vi "Tool.vi"() -> ()   [LabVIEW 2015]
uses:
  user32.dll
panel:
  in  "Tab":enum32{"MD5 Tool"}(tab)
  in  "Path":path caption="File Path"
  out "MD5 Checksum":string caption="String"
  in  "OK":bool
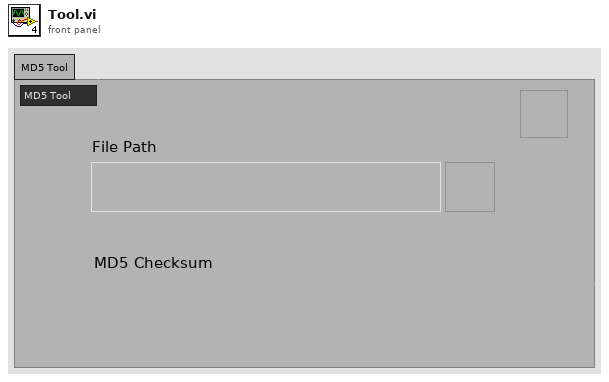
[diagram p1: front panel]
types:
  T1 = enum32{"invalid app kind", "Development System", "Run Time System", "Student Edition", "Embedded LabVIEW", "Evaluation", "Custom"}
  T2 = enum32{"Invalid", "Standard", "Closed", "Hidden", "Minimized", "Maximized"}
  T3 = cluster{"Core":cluster{"Current VI Reference":refnum<vi>, "Close Panel on Exit?":bool}, "Your Boolean data":bool, "Your string data":string}
  T4 = cluster{"Current VI Reference":refnum<vi>, "Close Panel on Exit?":bool}
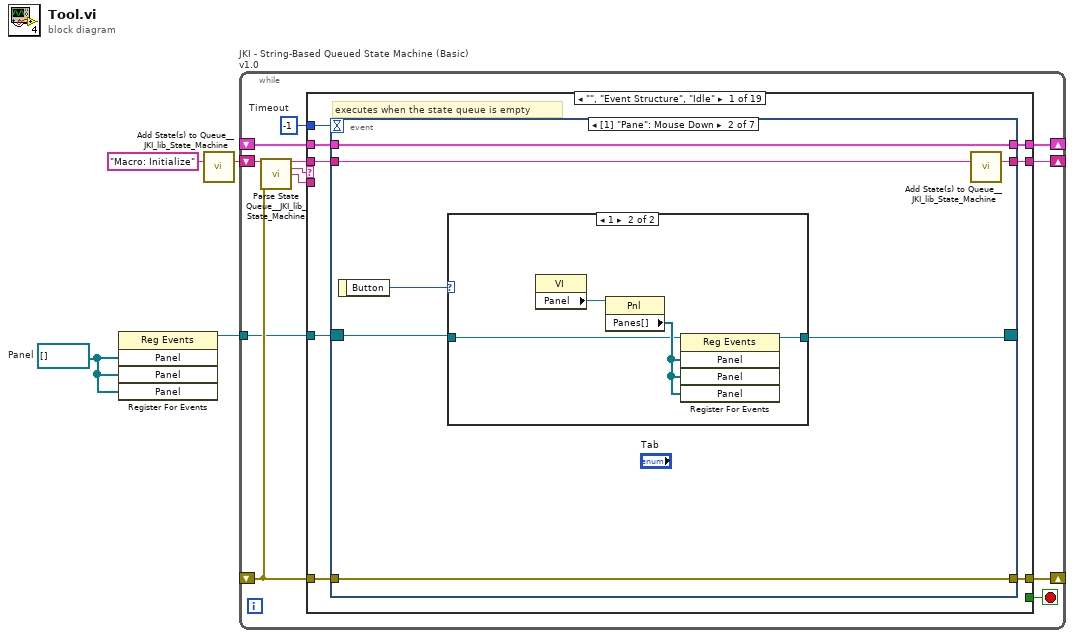
[diagram p0: block diagram]
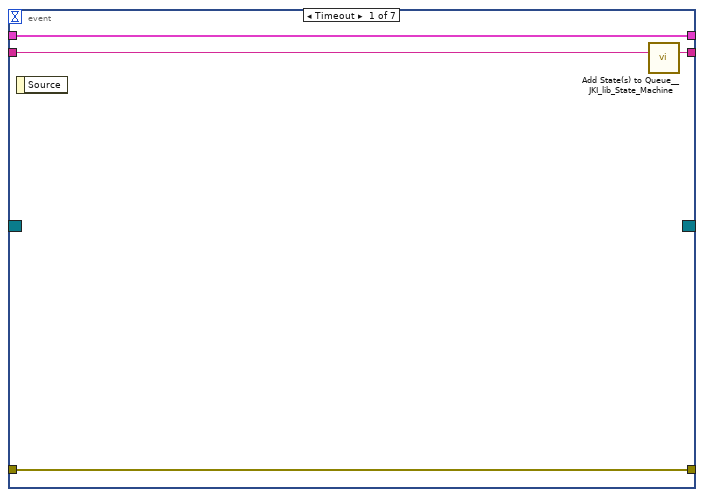
[diagram p2: hidden frame]
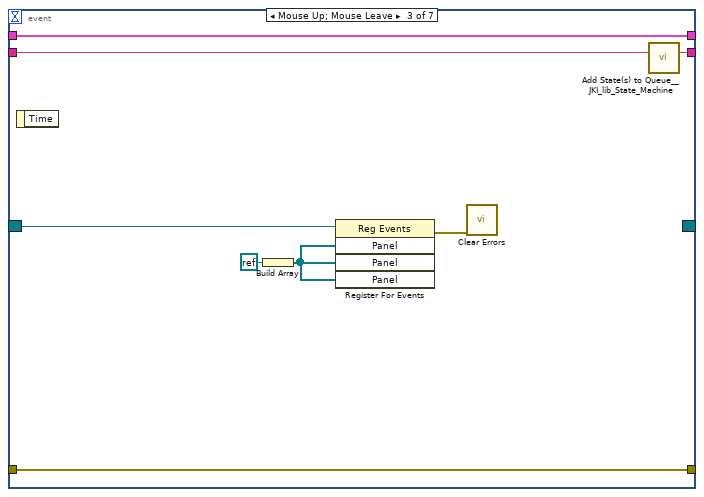
[diagram p4: hidden frame]
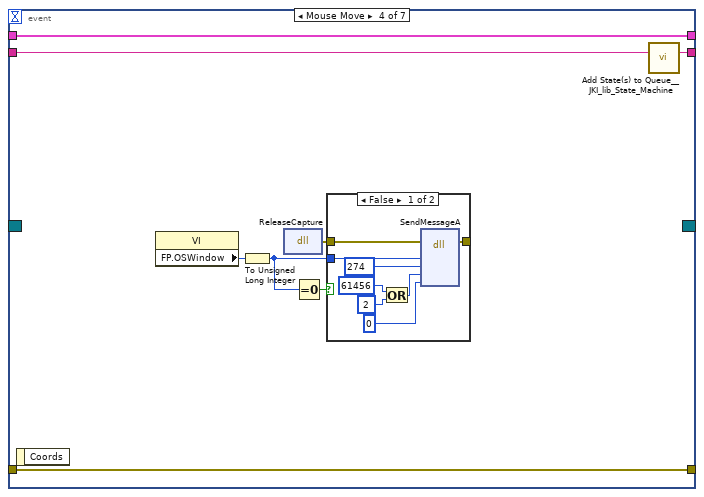
[diagram p5: hidden frame]
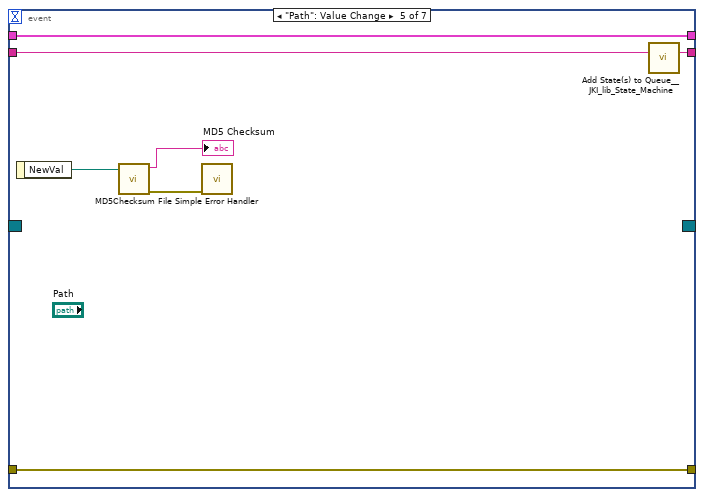
[diagram p7: hidden frame]
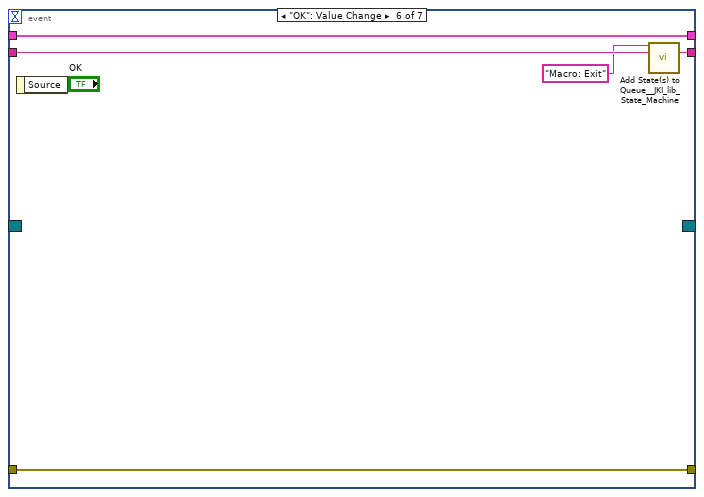
[diagram p8: hidden frame]
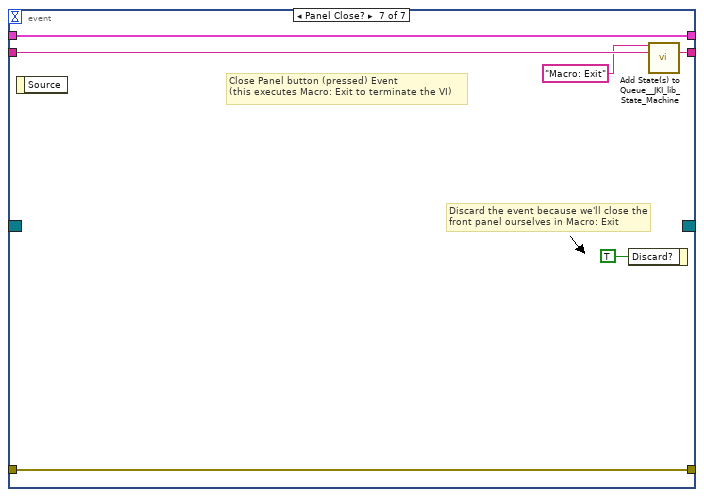
[diagram p9: hidden frame]
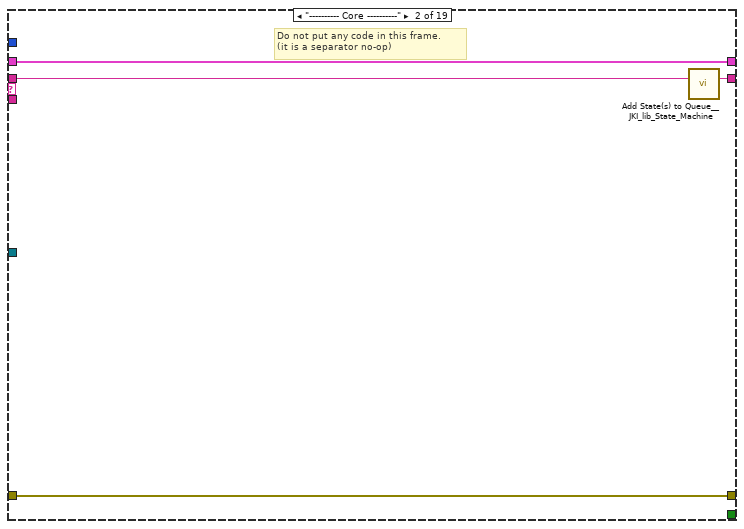
[diagram p10: hidden frame]
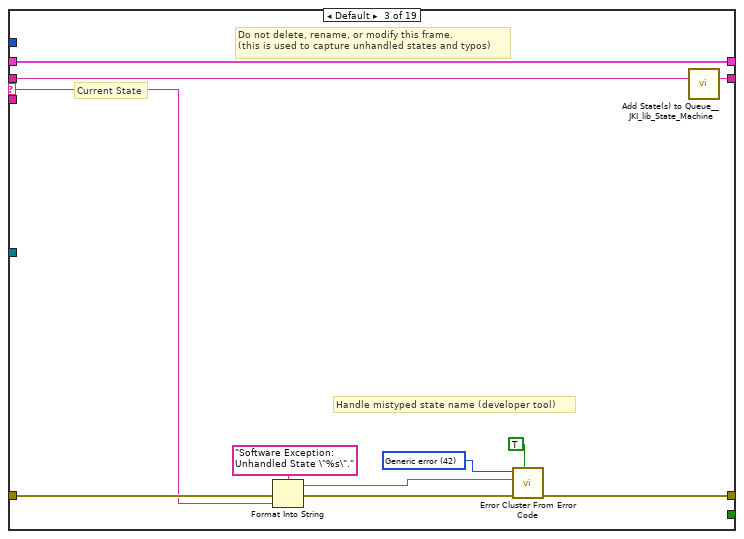
[diagram p11: hidden frame]
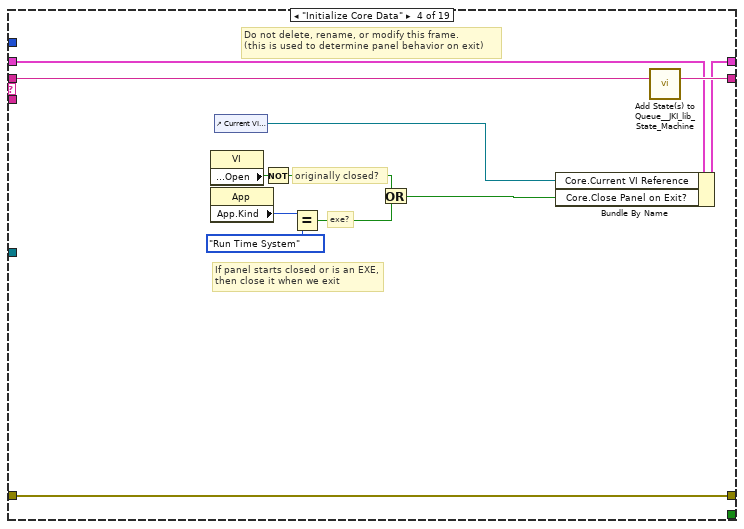
[diagram p12: hidden frame]
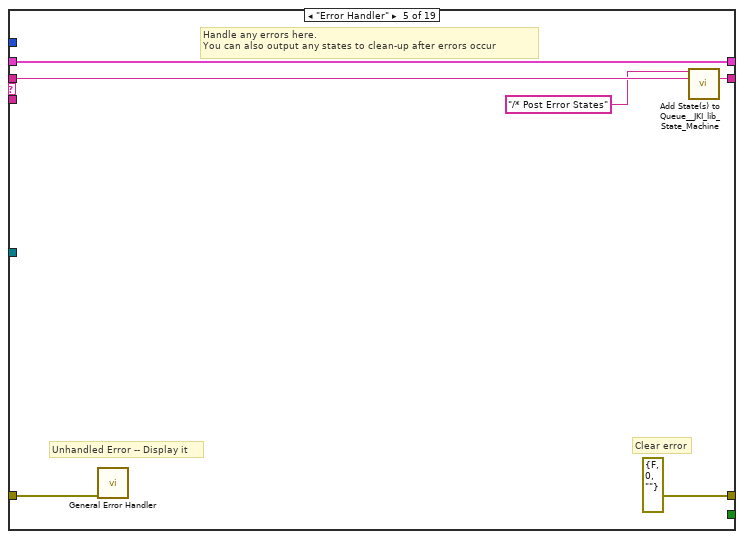
[diagram p13: hidden frame]
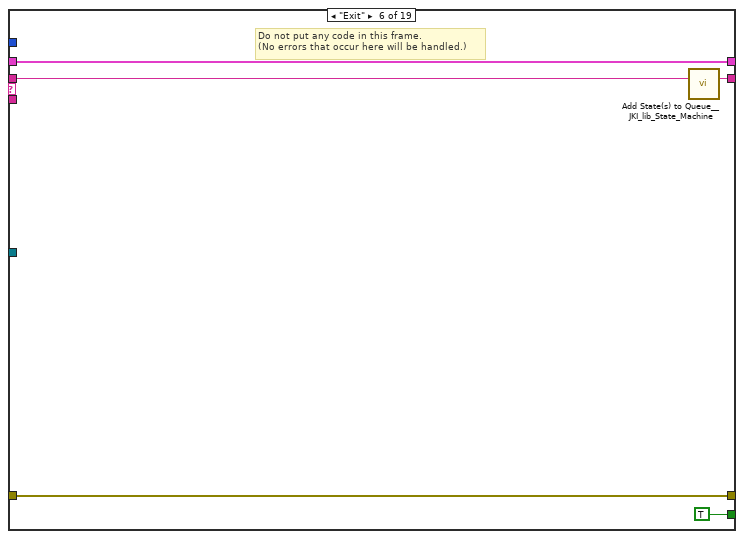
[diagram p14: hidden frame]
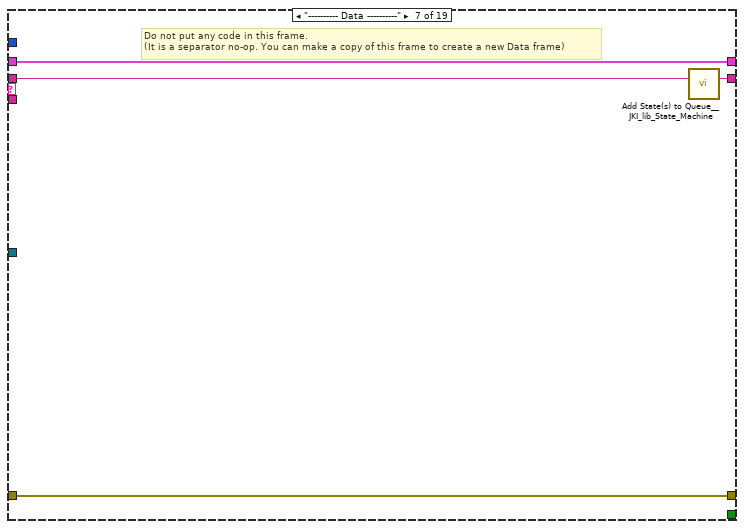
[diagram p15: hidden frame]
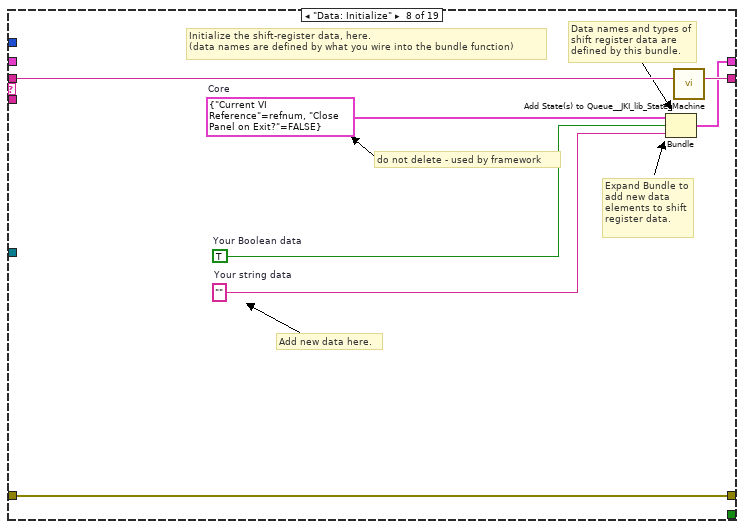
[diagram p16: hidden frame]
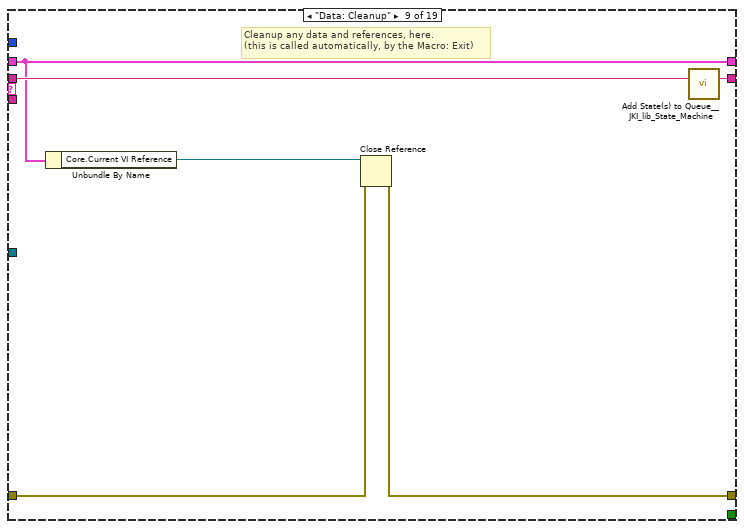
[diagram p17: hidden frame]
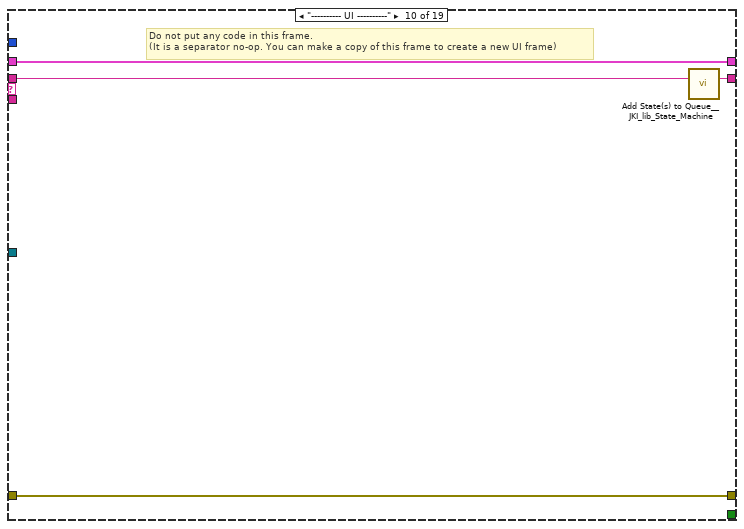
[diagram p18: hidden frame]
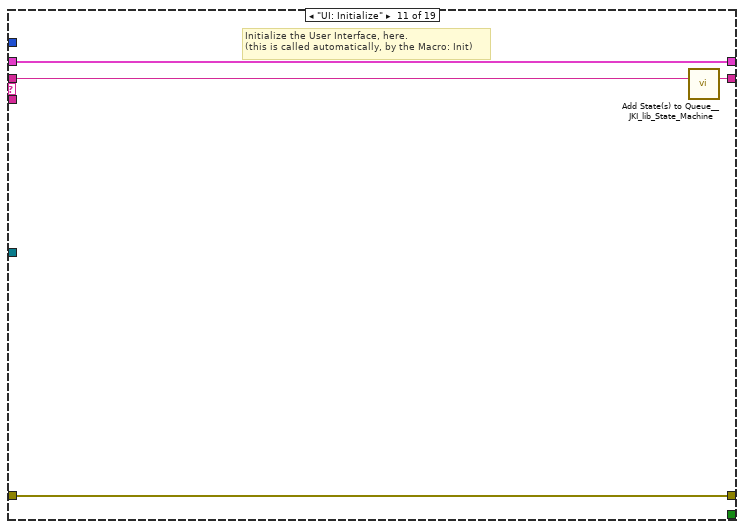
[diagram p19: hidden frame]
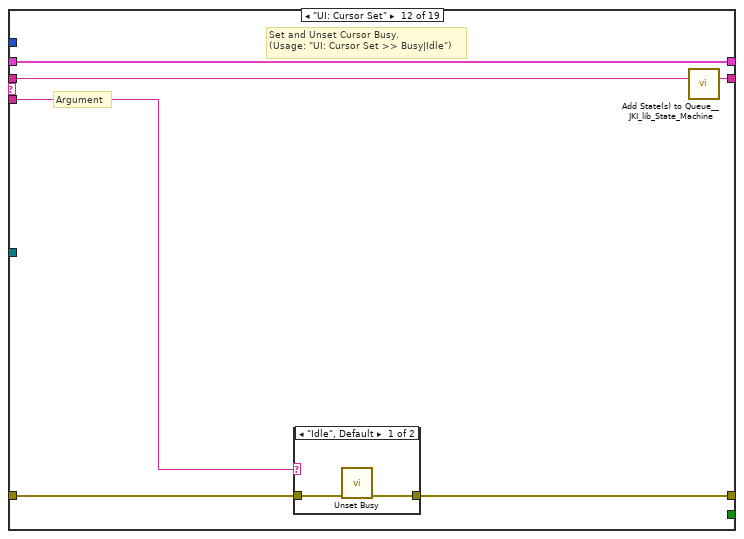
[diagram p20: hidden frame]
diagram:
  w2 = refnum<vi>[] []  # Panel
  n1 = register-events(w2, w2, w2) -> (reference out=w1:refnum<event-registration>)  [unwired: 2 in, 1 out]
  n2 = call <vilib>:"Add State(s) to Queue__JKI_lib_State_Machine.vi"("State(s) in (\"\")"="Macro: Initialize") -> ("States Out"=w4:string)  [unwired: 14 in]
  n3 = while "JKI - String-Based Queued State Machine (Basic) v1.0" {
    shift-right: [w9] -> _
    shift-left: _ -> [w8]
    shift-right: [w12] -> _
    shift-left: _ -> [w6]
    shift-right: [w11] -> _
    shift-left: w4 -> [w13]
    tunnel: w1 -> [w5]
    stop <- w10 stop-if-true
    w7 = -1  # Timeout
    n4 = call <vilib>:"Parse State Queue__JKI_lib_State_Machine.vi"("State Queue"=w13, "Error In (no error)"=w6) -> ("Remaining States"=w15:string, "Current State"=w16:string, "Arguments"=w14:string)  [unwired: 10 in, 1 out]
    n5 = case shown="\"\", \"Event Structure\", \"Idle\"" w16 {
      selector: w16 -> [_ _ w88 _ _ _ _ _ _ _ _ _ _ _ _ _ _ _ _]
      tunnel: w15 -> [w24 w87 w92 w110 w116 w121 w125 w132 w138 w142 w146 w152 w163 w189 w194 w204 w208 w212 w216]
      tunnel: w14 -> [_ _ _ _ _ _ _ _ _ _ _ w147 w157 _ _ _ _ _ _]
      tunnel: w8 -> [w22 w84 w90 w101 w113 w119 w122 _ w133 w139 w144 w150 w159 w186 w191 w201 w205 w209 w213]
      tunnel: [w21 w85 w94 w107 errorcluster {"status"=FALSE, "code"=0, "source"=""} ("error out") w118 w123 w129 w134 w140 w143 w148 w160 w187 w192 w202 w206 w210 w214] -> w12
      tunnel: w6 -> [w20 w85 w93 w107 w112 w118 w123 w129 w135 w140 w143 w149 w161 w187 w192 w202 w206 w210 w214]
      tunnel: [w23 w86 w91 w109 w115 w120 w124 w131 w137 w141 w145 w151 w162 w188 w193 w203 w207 w211 w215] -> w11
      tunnel: [_ _ _ _ _ TRUE _ _ _ _ _ _ _ _ _ _ _ _ _] -> w10
      tunnel: [w19 w84 w90 w108 w113 w119 w122 w130 w133 w139 w144 w150 w159 w186 w191 w201 w205 w209 w213] -> w9
      tunnel: w7 -> [w18 _ _ _ _ _ _ _ _ _ _ _ _ _ _ _ _ _ _]
      tunnel: w5 -> [w17 _ _ _ _ _ _ _ _ _ _ _ _ _ _ _ _ _ _]
      frame "", "Event Structure", "Idle" {
        # "executes when the state queue is empty"
        n6 = event shown="[1] \"Pane\": Mouse Down" {
          selector: w17 -> [_ w31 w41 _ _ _ _]
          dyn-events: [_ w29 _ _ _ _ _] -> _
          timeout: w18 -> [_ _ _ _ _ _ _]
          tunnel: w24 -> [w28 w35 w48 w56 w72 w77 w83]
          tunnel: [w27 w34 w47 w55 w71 w76 w82] -> w23
          tunnel: w22 -> [w25 w32 w45 w53 w69 w74 w80]
          tunnel: [w26 w33 w46 w54 w70 w75 w81] -> w21
          tunnel: w20 -> [w26 w33 w46 w54 w70 w75 w81]
          tunnel: [w25 w32 w45 w53 w69 w74 w80] -> w19
          event Timeout {
            n7 = event-data() -> ()  [unwired: 1 in, 1 out]
            n8 = call <vilib>:"Add State(s) to Queue__JKI_lib_State_Machine.vi"("State(s) in (\"\")"=w28) -> ("States Out"=w27:string)  [unwired: 14 in]
          }
          event Mouse Down {
            n9 = event-data() -> ("Button"=w30:u16)  [unwired: 1 in]
            n10 = case shown="1" w30 {
              tunnel: [w36 w37] -> w29
              tunnel: w31 -> [w36 w38]
              frame 0, Default {
              }
              frame 1 {
                n11 = property class="VI"() -> ("Panel"=w40:refnum<vi>)  [unwired: 2 in, 2 out]
                n12 = property class="Pnl"(reference=w40) -> ("Panes[]"=w39:refnum<vi>[])  [unwired: 1 in, 2 out]
                n13 = register-events(reference=w38, w39, w39, w39) -> (reference out=w37:refnum<event-registration>)  [unwired: 1 in, 1 out]
              }
            }
            n14 = call <vilib>:"Add State(s) to Queue__JKI_lib_State_Machine.vi"("State(s) in (\"\")"=w35) -> ("States Out"=w34:string)  [unwired: 14 in]
          }
          event Mouse Up; Mouse Leave {
            n15 = event-data() -> ()  [unwired: 1 in, 1 out]
            n16 = Build Array(refnum<k0> refnum) -> (w42:refnum<k0>[])
            n17 = register-events(reference=w41, w42, w42, w42) -> (error out=w43:errorcluster)  [unwired: 1 in, 1 out]
            n18 = call <vilib>:"Clear Errors.vi"("error in (no error)"=w43) -> ()  [unwired: 5 in, 2 out]
            n19 = call <vilib>:"Add State(s) to Queue__JKI_lib_State_Machine.vi"("State(s) in (\"\")"=w48) -> ("States Out"=w47:string)  [unwired: 14 in]
          }
          event Mouse Move {
            n20 = event-data() -> ()  [unwired: 1 in, 1 out]
            n21 = property class="VI"() -> ("FP.OSWindow"=w50:i32)  [unwired: 2 in, 2 out]
            n22 = To Unsigned Long Integer(number=w50) -> (unsigned 32bit integer=w49:u32)
            n23 = dll-call lib="user32.dll" fn="ReleaseCapture"() -> (error out=w52:errorcluster)  [unwired: 3 in, 2 out]
            n24 = Equal To 0?(x=w49) -> (x = 0?=w51:bool)
            n25 = case shown="False" w51 {
              tunnel: [w64 w65] -> _
              tunnel: w52 -> [w63 w65]
              tunnel: w49 -> [w62 _]
              frame False {
                n26 = Or(x=u32 61456 ("wMsg"), y=u32 2 ("wMsg")) -> (x .or. y?=w58:u32)
                n27 = dll-call lib="user32.dll" fn="SendMessageA"(error in=w63, "hWnd"=w62, "wMsg"=u32 274, "wParam"=w58, "lParam"=0) -> (error out=w64:errorcluster)  [unwired: 6 in, 2 out]
              }
              frame True {
              }
            }
            n28 = call <vilib>:"Add State(s) to Queue__JKI_lib_State_Machine.vi"("State(s) in (\"\")"=w56) -> ("States Out"=w55:string)  [unwired: 14 in]
          }
          event "Path": Value Change {
            n29 = event-data() -> ("NewVal"=w66:path)  [unwired: 1 in]
            n30 = call <vilib>:"MD5Checksum File.vi"("Path"=w66) -> ("error out"=w67:errorcluster, "MD5 message-digest"=→"MD5 Checksum":string)  [unwired: 9 in]
            n31 = call <vilib>:"Simple Error Handler.vi"("error in (no error)"=w67) -> ()  [unwired: 4 in, 5 out]
            n32 = call <vilib>:"Add State(s) to Queue__JKI_lib_State_Machine.vi"("State(s) in (\"\")"=w72) -> ("States Out"=w71:string)  [unwired: 14 in]
          }
          event "OK": Value Change {
            n33 = event-data() -> ()  [unwired: 1 in, 1 out]
            n34 = call <vilib>:"Add State(s) to Queue__JKI_lib_State_Machine.vi"("State(s) in Front (\"\")"="Macro: Exit", "State(s) in (\"\")"=w77) -> ("States Out"=w76:string)  [unwired: 13 in]
          }
          event Panel Close? {
            # "Discard the event because we'll close the front panel ourselves in Macro: Exit"
            # "Close Panel button (pressed) Event\n(this executes Macro: Exit to terminate the VI)"
            n35 = event-data() -> ()  [unwired: 1 in, 1 out]
            n36 = event-data("Discard?"=TRUE) -> ()  [unwired: 1 in, 1 out]
            n37 = call <vilib>:"Add State(s) to Queue__JKI_lib_State_Machine.vi"("State(s) in Front (\"\")"="Macro: Exit", "State(s) in (\"\")"=w83) -> ("States Out"=w82:string)  [unwired: 13 in]
          }
        }
      }
      frame "---------- Core ----------" {
        # "Do not put any code in this frame.\n(it is a separator no-op)"
        n38 = call <vilib>:"Add State(s) to Queue__JKI_lib_State_Machine.vi"("State(s) in (\"\")"=w87) -> ("States Out"=w86:string)  [unwired: 14 in]
      }
      frame Default {
        w97 = 42 items=["No error", "Argument error", "Memory is full", "Out of zone", "End of file", "File already open", "Generic file I/O error", "File not found", "File permission error", "Disk is full", "Duplicate path", "Too many files open", "System feature not enabled", "Resource file not found", "Cannot add resource", "Resource not found", "Image not found", "Image memory error", "Pen does not exist", "Config type invalid", "Config token not found", "Config parse error", "Config memory error", "Bad external code format", "Bad external code offset", "External code not present", "Null window", "Destroy window error", "Null menu", "Print aborted", "Bad print record", "Print driver error", "Windows error during printing", "Memory error during printing", "Print dialog error", "Generic print error", "Invalid device refnum", "Device not found", "Device parameter error", "Device unit error", "Cannot open device", "Device call aborted", "Generic error", "Cancelled by user", "Object ID too low", "Object ID too high", "Object not in heap", "Unknown heap", "Unknown object (invalid DefProc)", "Unknown object (DefProc not in table)", "Message out of range", "Invalid (null) method", "Unknown message", "Manager call not supported", "Bad address", "Network operation in progress", "Network operation timed out", "Connection is busy", "Network attribute not supported", "Network error", "Address in use", "System out of memory", "Connection aborted", "Connection refused", "Not connected", "Already connected", "Connection closed", "Initialization error (interapplication manager)", "Bad occurrence", "Wait on unbound occurrence handler", "Occurrence queue overflow", "Datalog type conflict", "Unused", "Unrecognized type (interapplication manager)", "Memory corrupt", "Failed to make temporary DLL", "Old CIN version", "Drag socket not found", "Failed to load drop-object", "Failed to register OLE object", "Failed to release OLE object", "Format specifier type mismatch", "Unknown format specifier", "Too few format specifiers", "Too many format specifiers", "Scan failed", "Newer CIN version", "Error converting to variant", "Runtime menu error", "Password tampered", "Variant attribute not found", "Incompatible variant data type", "Event data is not available", "Event Store is not present", "Occurrence is not found", "Event Queue is not created", "Event info is not available", "Refnum passed is NULL", "Error retrieving Class GUID", "Error retrieving CoClass GUID", "Error retrieving TypeLib GUID.", "Bad built application magic bytes.", "Specific driver is different from the specific driver associated with the Logical Name.", "There is no session opened to the class driver.", "Max Error", "MAX - Error with config objects", "MAX - Error loading configuration", "MAX - Group not supported"]
        # "Current State"
        # "Do not delete, rename, or modify this frame.\n(this is used to capture unhandled states and typos)"
        # "Handle mistyped state name (developer tool)"
        n39 = Format Into String(format string="Software Exception: Unhandled State \"%s\"." ("message"), error in=w93, w88) -> (resulting string=w96:string, error out=w95:errorcluster)  [unwired: 1 in]
        n40 = call <vilib>:"Error Cluster From Error Code.vi"("show call chain? (False)"=TRUE, "error in (no error)"=w95, "error message (\"\")"=w96, "error code (0)"=w97) -> ("error out"=w94:errorcluster)  [unwired: 5 in]
        n41 = call <vilib>:"Add State(s) to Queue__JKI_lib_State_Machine.vi"("State(s) in (\"\")"=w92) -> ("States Out"=w91:string)  [unwired: 14 in]
      }
      frame "Initialize Core Data" {
        # "Do not delete, rename, or modify this frame.\n(this is used to determine panel behavior on exit)"
        # "originally closed?"
        # "exe?"
        # "If panel starts closed or is an EXE, then close it when we exit"
        n42 = property class="VI"() -> ("Front Panel.Open"=w106:bool)  [unwired: 2 in, 2 out]
        n43 = property class="App"() -> ("App.Kind"=w105:T1)  [unwired: 2 in, 2 out]
        n44 = control-ref of="Current VI Reference"() -> (w99:refnum<vi>)
        n45 = Not(x=w106) -> (.not. x?=w103:bool)
        n46 = Equal?(x=w105, y=T1."Run Time System" ("Application:Kind")) -> (x = y?=w102:bool)
        n47 = Or(x=w103, y=w102) -> (x .or. y?=w100:bool)
        n48 = Bundle By Name(cluster=w101, "Core.Current VI Reference"=w99, "Core.Close Panel on Exit?"=w100) -> (w108:T3)
        n49 = call <vilib>:"Add State(s) to Queue__JKI_lib_State_Machine.vi"("State(s) in (\"\")"=w110) -> ("States Out"=w109:string)  [unwired: 14 in]
      }
      frame "Error Handler" {
        # "Unhandled Error -- Display it"
        # "Handle any errors here.\nYou can also output any states to clean-up after errors occur"
        # "Clear error"
        n50 = call <vilib>:"General Error Handler.vi"("error in (no error)"=w112) -> ()  [unwired: 10 in, 5 out]
        n51 = call <vilib>:"Add State(s) to Queue__JKI_lib_State_Machine.vi"("State(s) in Front (\"\")"="/* Post Error States", "State(s) in (\"\")"=w116) -> ("States Out"=w115:string)  [unwired: 13 in]
      }
      frame "Exit" {
        # "Do not put any code in this frame.\n(No errors that occur here will be handled.)"
        n52 = call <vilib>:"Add State(s) to Queue__JKI_lib_State_Machine.vi"("State(s) in (\"\")"=w121) -> ("States Out"=w120:string)  [unwired: 14 in]
      }
      frame "---------- Data ----------" {
        # "Do not put any code in this frame.\n(It is a separator no-op. You can make a copy of this frame to create a new Data frame)"
        n53 = call <vilib>:"Add State(s) to Queue__JKI_lib_State_Machine.vi"("State(s) in (\"\")"=w125) -> ("States Out"=w124:string)  [unwired: 14 in]
      }
      frame "Data: Initialize" {
        w126 = T4 {"Current VI Reference"=refnum, "Close Panel on Exit?"=FALSE}  # Core
        w128 = TRUE  # Your Boolean data
        w127 = ""  # Your string data
        # "do not delete - used by framework"
        # "Expand Bundle to add new data elements to shift register data."
        # "Add new data here."
        # "Data names and types of shift register data are defined by this bundle."
        # "Initialize the shift-register data, here.\n(data names are defined by what you wire into the bundle function)"
        n54 = Bundle("Core"=w126, "Your Boolean data"=w128, "Your string data"=w127) -> (w130:T3)  [unwired: 1 in]
        n55 = call <vilib>:"Add State(s) to Queue__JKI_lib_State_Machine.vi"("State(s) in (\"\")"=w132) -> ("States Out"=w131:string)  [unwired: 14 in]
      }
      frame "Data: Cleanup" {
        # "Cleanup any data and references, here.\n(this is called automatically, by the Macro: Exit)"
        n56 = Unbundle By Name(w133) -> ("Core.Current VI Reference"=w136:refnum<vi>)
        n57 = Close Reference(reference=w136, error in (no error)=w135) -> (error out=w134:errorcluster)
        n58 = call <vilib>:"Add State(s) to Queue__JKI_lib_State_Machine.vi"("State(s) in (\"\")"=w138) -> ("States Out"=w137:string)  [unwired: 14 in]
      }
      frame "---------- UI ----------" {
        # "Do not put any code in this frame.\n(It is a separator no-op. You can make a copy of this frame to create a new UI frame)"
        n59 = call <vilib>:"Add State(s) to Queue__JKI_lib_State_Machine.vi"("State(s) in (\"\")"=w142) -> ("States Out"=w141:string)  [unwired: 14 in]
      }
      frame "UI: Initialize" {
        # "Initialize the User Interface, here.\n(this is called automatically, by the Macro: Init)"
        n60 = call <vilib>:"Add State(s) to Queue__JKI_lib_State_Machine.vi"("State(s) in (\"\")"=w146) -> ("States Out"=w145:string)  [unwired: 14 in]
      }
      frame "UI: Cursor Set" {
        # "Argument"
        # "Set and Unset Cursor Busy.\n(Usage: \"UI: Cursor Set >> Busy|Idle\")"
        n61 = case shown="\"Idle\", Default" w147 {
          tunnel: w149 -> [w154 w156]
          tunnel: [w153 w155] -> w148
          frame "Idle", Default {
            n62 = call <vilib>:"Unset Busy.vi"("error in (no error)"=w154) -> ("error out"=w153:errorcluster)  [unwired: 10 in]
          }
          frame "Busy" {
            n63 = call <vilib>:"Set Busy.vi"("error in (no error)"=w156) -> ("error out"=w155:errorcluster)  [unwired: 9 in, 1 out]
          }
        }
        n64 = call <vilib>:"Add State(s) to Queue__JKI_lib_State_Machine.vi"("State(s) in (\"\")"=w152) -> ("States Out"=w151:string)  [unwired: 14 in]
      }
      frame "UI: Front Panel State" {
        # "Argument"
        # "Set Front Panel Open or Closed\n(Usage: \"UI: Front Panel State >> Open|Close\")"
        n65 = Unbundle By Name(w159) -> ("Core.Current VI Reference"=w158:refnum<vi>)
        n66 = case shown="\"Open\", Default" w157 {
          tunnel: w161 -> [w167 w180]
          tunnel: [w169 w181] -> w160
          tunnel: w158 -> [w168 w178]
          frame "Open", Default {
            n67 = property class="VI"(reference=w168, error in=w167) -> (reference out=w165:refnum<vi>, error out=w166:errorcluster, "Front Panel.Open"=w164:bool)
            n68 = case shown="False" w164 {
              tunnel: [w172 w175] -> w169
              tunnel: w166 -> [w171 w175]
              tunnel: w165 -> [w170 _]
              frame False {
                n69 = invoke class="VI" method="FP.Open"(reference=w170, error in=w171, "Activate"=TRUE, "State"=T2."Standard") -> (error out=w172:errorcluster)  [unwired: 1 in, 4 out]
              }
              frame True {
              }
            }
          }
          frame "Close" {
            n70 = property class="VI"(reference=w178, error in=w180) -> (reference out=w177:refnum<vi>, error out=w179:errorcluster, "Front Panel.Open"=w176:bool)
            n71 = case shown="True" w176 {
              tunnel: [w182 w185] -> w181
              tunnel: w179 -> [w182 w184]
              tunnel: w177 -> [_ w183]
              frame False {
              }
              frame True {
                n72 = invoke class="VI" method="FP.Close"(reference=w183, error in=w184) -> (error out=w185:errorcluster)  [unwired: 1 in, 2 out]
              }
            }
          }
        }
        n73 = call <vilib>:"Add State(s) to Queue__JKI_lib_State_Machine.vi"("State(s) in (\"\")"=w163) -> ("States Out"=w162:string)  [unwired: 14 in]
      }
      frame "---------- Macro ----------" {
        # "Do not put any code in this frame.\n(It is a separator no-op. You can make a copy of this frame to create a new Macro frame)"
        n74 = call <vilib>:"Add State(s) to Queue__JKI_lib_State_Machine.vi"("State(s) in (\"\")"=w189) -> ("States Out"=w188:string)  [unwired: 14 in]
      }
      frame "Macro: Initialize" {
        w190 = "Data: Initialize\nInitialize Core Data\nUI: Initialize\nUI: Front Panel State >> Open"  # Data: Initialize Initialize Core Data UI: Initialize UI: Front Panel State >> Open
        # "Initialization Macro\n(This is called once, when the VI starts)"
        n75 = call <vilib>:"Add State(s) to Queue__JKI_lib_State_Machine.vi"("State(s) in Front (\"\")"=w190, "State(s) in (\"\")"=w194) -> ("States Out"=w193:string)  [unwired: 13 in]
      }
      frame "Macro: Exit" {
        # "Exit Macro\n(This is called once, when the VI exits)"
        n76 = Unbundle By Name(w201) -> ("Core.Close Panel on Exit?"=w200:bool)
        n77 = Select(t="UI: Front Panel State >> Close", s=w200, f="") -> (s? t:f=w197:string)
        n78 = call <vilib>:"Add State(s) to Queue__JKI_lib_State_Machine.vi"("State(s) in (\"\")"=w197, "State(s) at Back (\"\")"="Data: Cleanup\nExit") -> ("States Out"=w195:string)  [unwired: 13 in]
        n79 = call <vilib>:"Add State(s) to Queue__JKI_lib_State_Machine.vi"("State(s) in Front (\"\")"=w195, "State(s) in (\"\")"=w204) -> ("States Out"=w203:string)  [unwired: 13 in]
      }
      frame "---------- New Category ----------" {
        # "Template Separator\n(You can make a copy of, or modify, this frame)"
        n80 = call <vilib>:"Add State(s) to Queue__JKI_lib_State_Machine.vi"("State(s) in (\"\")"=w208) -> ("States Out"=w207:string)  [unwired: 14 in]
      }
      frame "New Category: 1" {
        # "Your code here.\n(You can make a copy of, or modify, this frame)"
        n81 = call <vilib>:"Add State(s) to Queue__JKI_lib_State_Machine.vi"("State(s) in (\"\")"=w212) -> ("States Out"=w211:string)  [unwired: 14 in]
      }
      frame "New Category: 2" {
        # "Your code here.\n(You can make a copy of, or modify, this frame)"
        n82 = call <vilib>:"Add State(s) to Queue__JKI_lib_State_Machine.vi"("State(s) in (\"\")"=w216) -> ("States Out"=w215:string)  [unwired: 14 in]
      }
    }
  }
